vi "添加设备.vi"(7 "模式":enum16{"新建设备", "编辑设备"}(ring), 8 "错误输出":errorcluster, 11 "探头属性 i":T1) -> (0 "error out":errorcluster, 1 "附加信息":string, 2 "输出有效？":bool=TRUE, 3 "探头属性 o":T1)   [LabVIEW 2017]
doc: "修改信息时 : 输入完整信息 ,\n新建时 : 输入空常量 ."
uses:
  <vilib>/Utility/miscctls.llb/LVSelectionTypeDef.ctl
  df94b285-9738-4c66-b3c8-f98dc0b9297b.vi
  c5779a91-24a2-4c03-8a90-ef35a31279a1.vi
panel:
  out "改串口地址?":bool
  out "前缀":enum16{"Net", "Serial"}(ring)
  out "专用标志-首次 '端口值改变' 事件":bool=TRUE
  in  "设置系数":bool
  in  "类型":enum16{"网络探头", "串口探头"}(ring)
  in  "超时":i32
  out "已保存的探头号":u16[](array[numeric])
  in  "标题":string
  out "提示语 2":string
  in  "探头备注":string
  out "提示语":string
  in  "探头名称":string caption="探头名称 *"
  in  "取消":bool
  in  "确定":bool
  in  "地址":string caption="探头 *"
  in  "端口":u16 caption="探头号 *" min=1 max=255
  out "有效名称？":bool
  out "有效地址？":bool
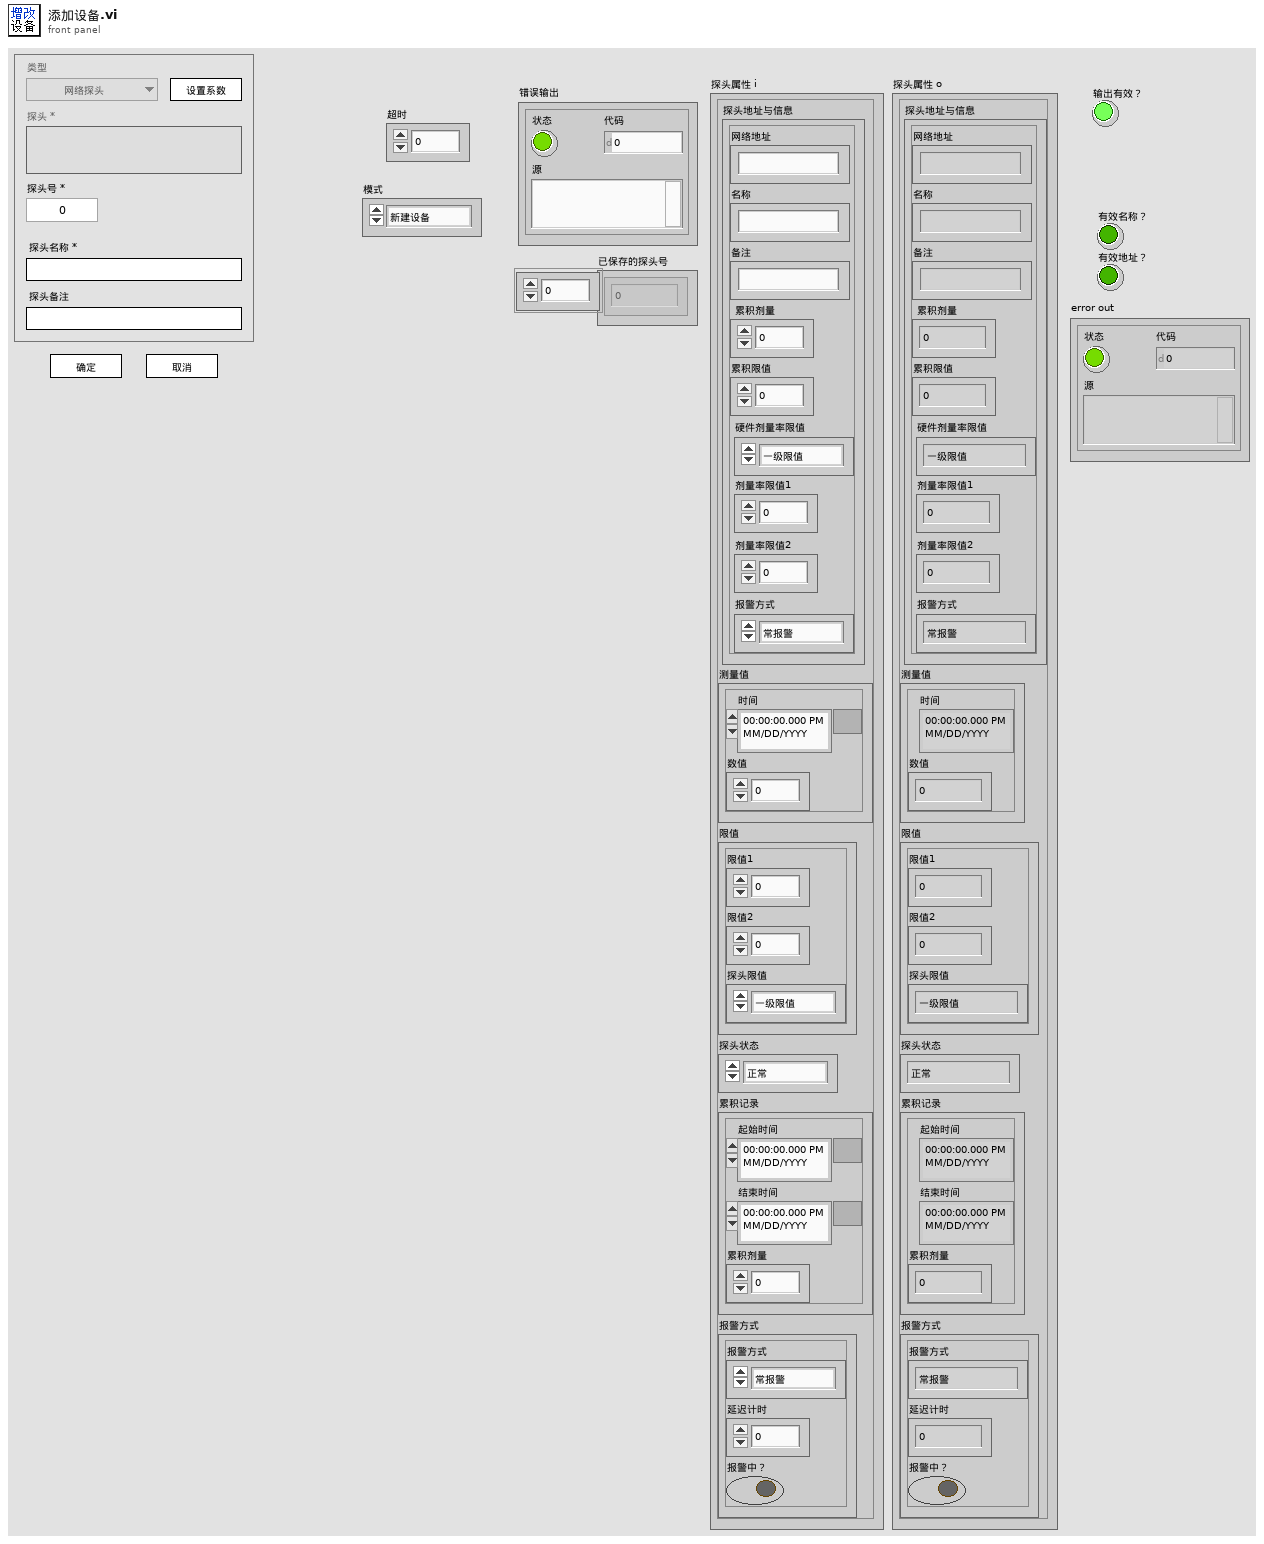
[diagram p1: front panel]
types:
  T1 = typedef "探头属性.ctl" = cluster{"探头地址与信息":T2, "测量值":T5, "限值":T6, "探头状态":T7, "累积记录":T8, "报警方式":T9}
  T2 = typedef "探测器信息.ctl" = cluster{"网络地址":string, "名称":string, "备注":string, "累积剂量":dbl, "累积限值":dbl, "硬件剂量率限值":T3, "剂量率限值1":dbl, "剂量率限值2":dbl, "报警方式":T4}
  T3 = typedef "探头剂量率限值选择.ctl" = enum16{"一级限值", "二级限值"}
  T4 = typedef "报警方式选择.ctl" = enum16{"常报警", "自动静音", "手动静音"}
  T5 = typedef "测量值.ctl" = cluster{"时间":timestamp, "数值":dbl}
  T6 = typedef "剂量率限值.ctl" = cluster{"限值1":dbl, "限值2":dbl, "探头限值":T3}
  T7 = typedef "探头状态.ctl" = enum16{"正常", "离线", "禁用", "一级报警", "二级报警", "累积报警"}
  T8 = typedef "单条累积记录.ctl" = cluster{"起始时间":timestamp, "结束时间":timestamp, "累积剂量":dbl}
  T9 = typedef "报警方式.ctl" = cluster{"报警方式":T4, "延迟计时":u16, "报警中？":bool}
  T10 = enum32{"Invalid", "Standard", "Closed", "Hidden", "Minimized", "Maximized"}
  T11 = typedef "DB动作与数据.ctl" = cluster{"动作类型":T12, "输入数据":variant}
  T12 = typedef "DB动作类型.ctl" = enum16{"DB-文件初始化+连接", "DB-断开连接", "DB-结构初始化", "DB-加载设备", "DB-检查连接状态", "设备-登记新设备+数据表", "设备-删除设备", "设备-修改网址", "设备-修改名称+转移数据", "设备-修改备注", "设备-修改限值", "设备-累积校准", "设备-重排", "数据-获取全部", "数据-删除数据", "数据-写改累积记录+改累积剂量", "读变量-全部设备"}
  T13 = typedef "串口配置.ctl" = cluster{"COM口":refnum<visa-resource-name>, "波特率":enum16{"9600", "19200"}, "探头地址(U8)":u8}
  T14 = typedef "探头系数.ctl" = cluster{"N1":u16, "N2":u16}
  T15 = typedef "串口模块输入.ctl" = cluster{"串口动作类型":T16, "串口配置":T13, "数据输入":variant}
  T16 = typedef "串口动作类型.ctl" = enum16{"读测量值", "设置报警值", "设置地址", "设置系数", "广播修改波特率", "关闭串口"}
  T17 = enum8{"Enabled", "Disabled", "Disabled and Grayed Out"}
  T18 = typedef "LVSelectionTypeDef.ctl" = cluster{"Selection Start":u32, "Selection End":u32}
  T19 = typedef "簇-输入.ctl" = cluster{"配置文件动作":T20, "数据输入":variant}
  T20 = typedef "枚举-配置文件动作.ctl" = enum16{"初始化加载配置", "读取配置", "写入-屏幕键盘", "写入-静音延迟", "写入-主要探头类型", "写入-串口配置", "写入-累积定时", "写入-导出定时", "保存配置到文件"}
  T21 = typedef "簇-配置文件内容.ctl" = cluster{"调试模式？":bool, "屏幕键盘？":bool, "软件版本":string, "静音延迟 s":u16, "主要探头类型":T22, "串口配置":cluster{"COM口":refnum<visa-resource-name>, "波特率":enum16{"9600", "19200"}, "读写超时ms":i16, "丢包判定次数":i16}, "定时配置-累积分段":T23, "定时配置-自动导出":cluster{"定时配置-自动导出":T23, "分别导出?":bool}}
  T22 = typedef "枚举-主要探头类型.ctl" = enum16{"网络探头", "串口探头"}
  T23 = typedef "簇-定时配置.ctl" = cluster{"定时模式":enum16{"绝对时间", "相对时间"}, "单位":enum16{"年", "月", "日", "时", "分"}, "间隔":u8, "目标时刻":timestamp}
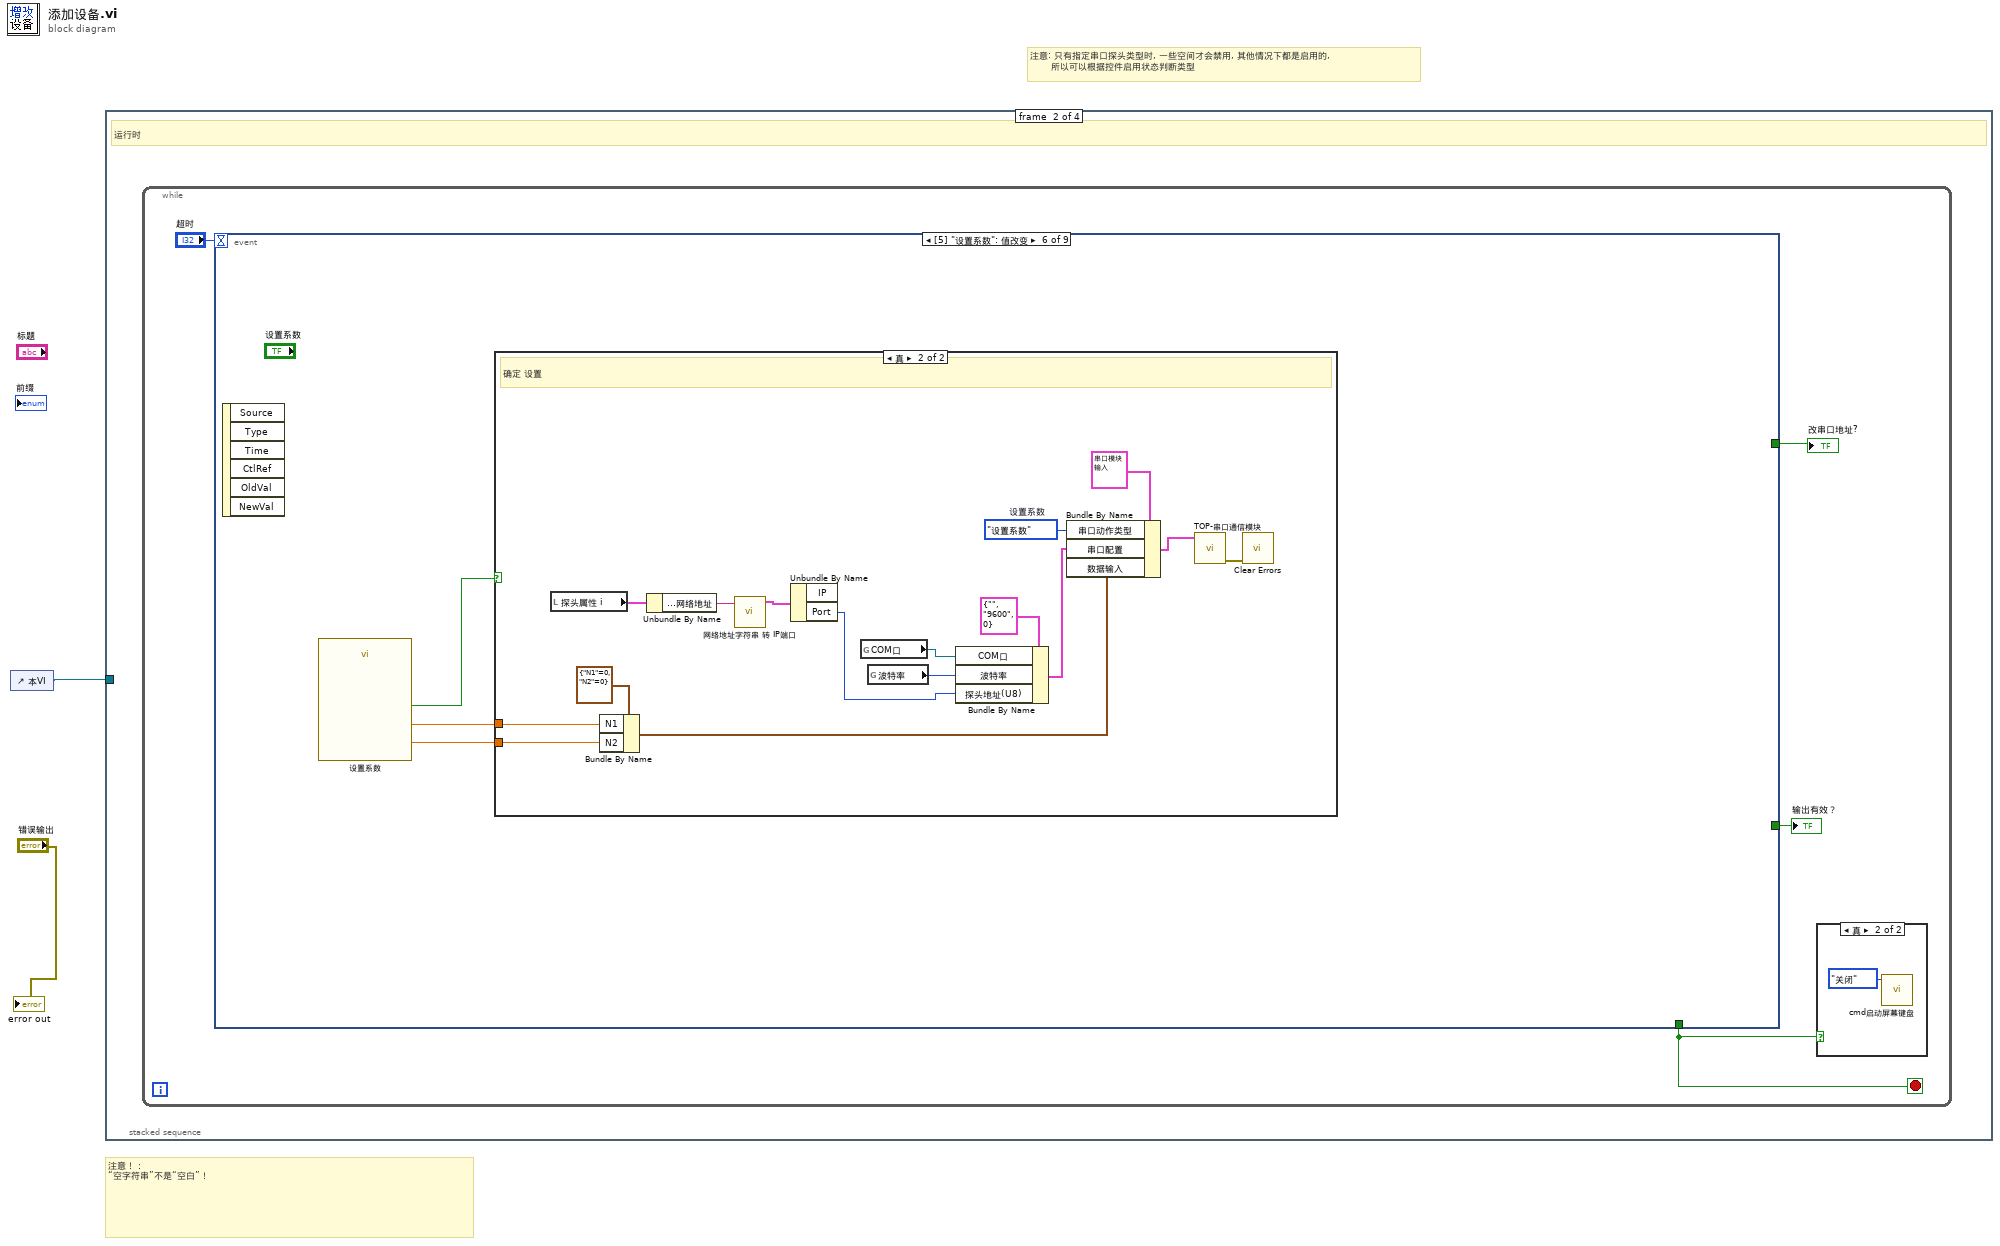
[diagram p0: block diagram]
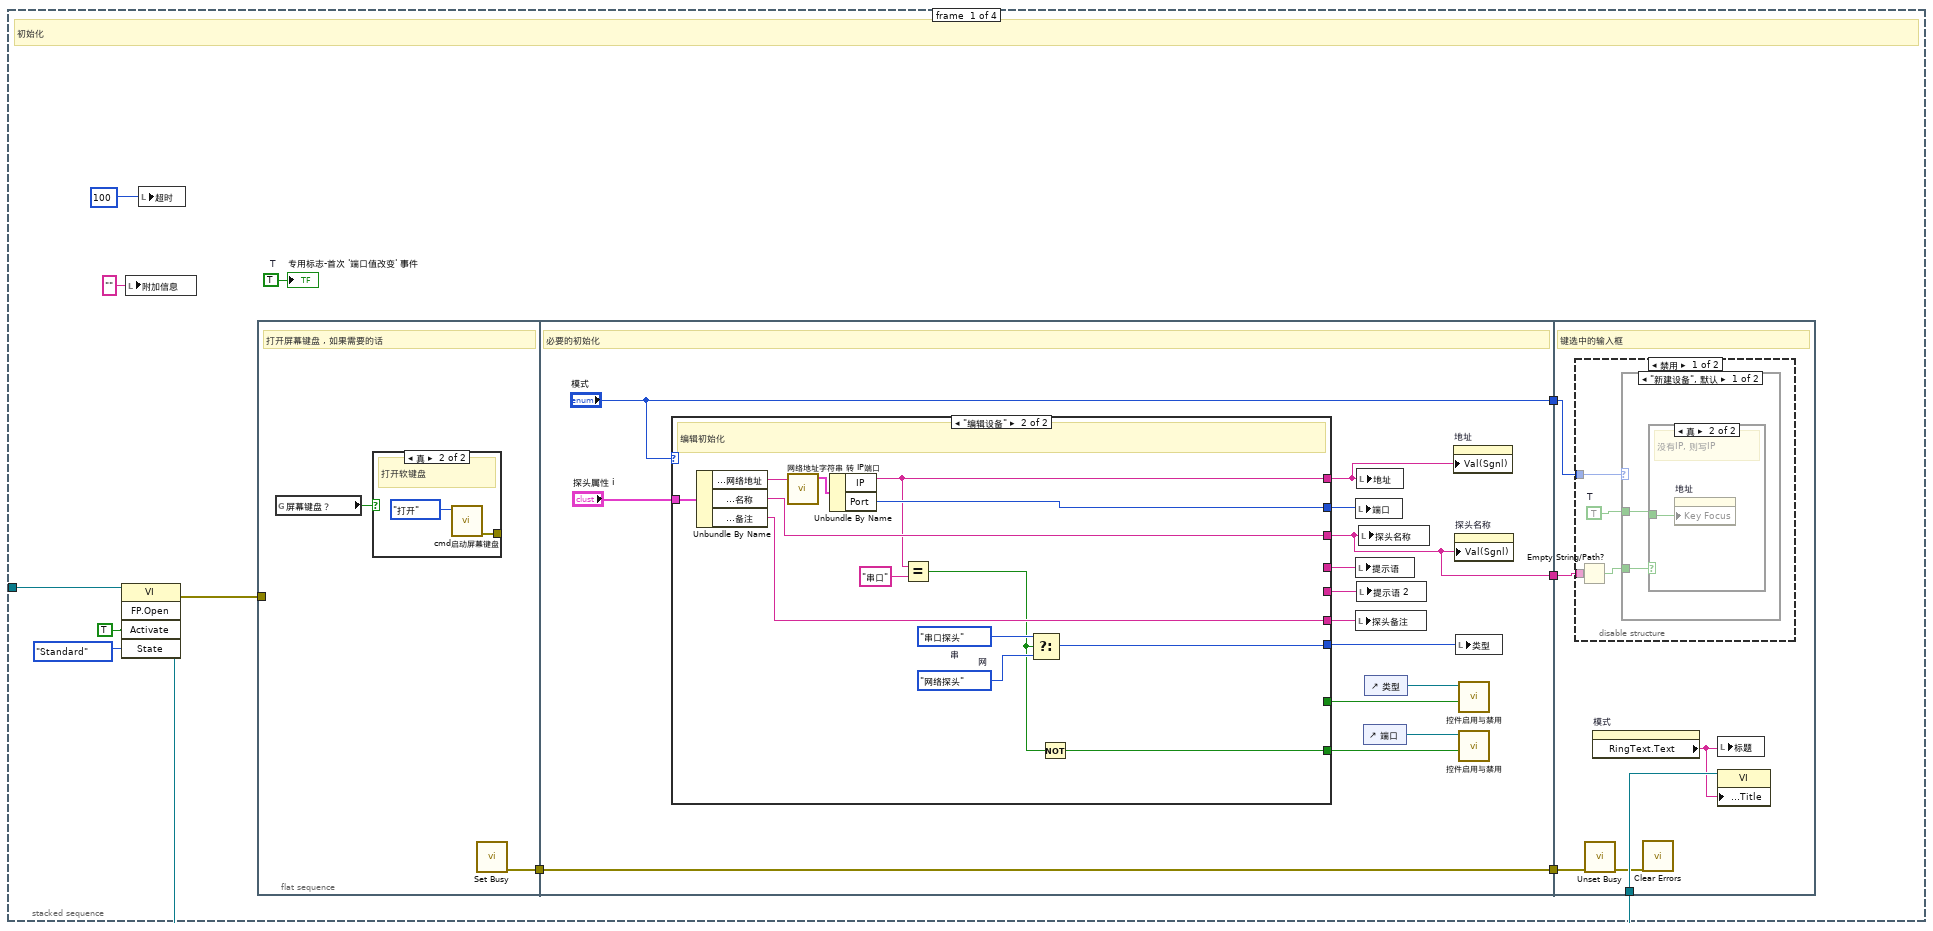
[diagram p2: hidden frame]
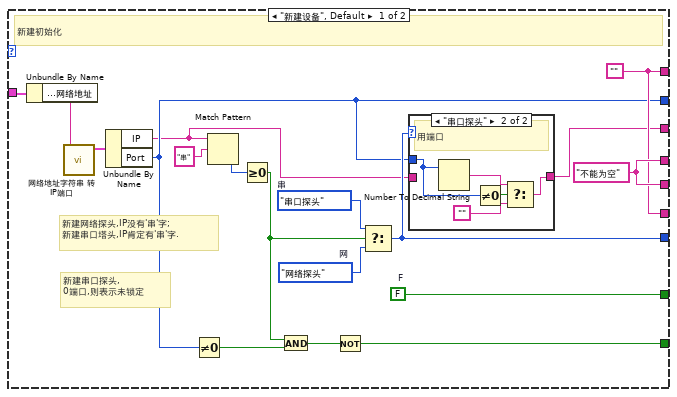
[diagram p4: hidden frame]
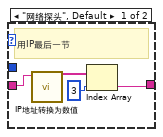
[diagram p5: hidden frame]
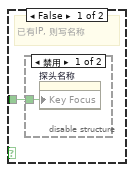
[diagram p6: hidden frame]
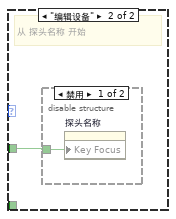
[diagram p8: hidden frame]
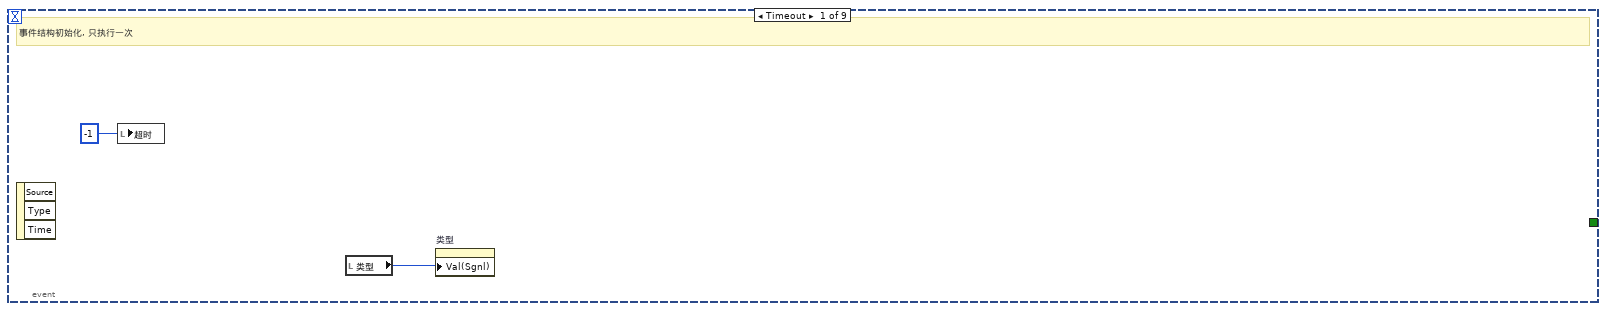
[diagram p12: hidden frame]
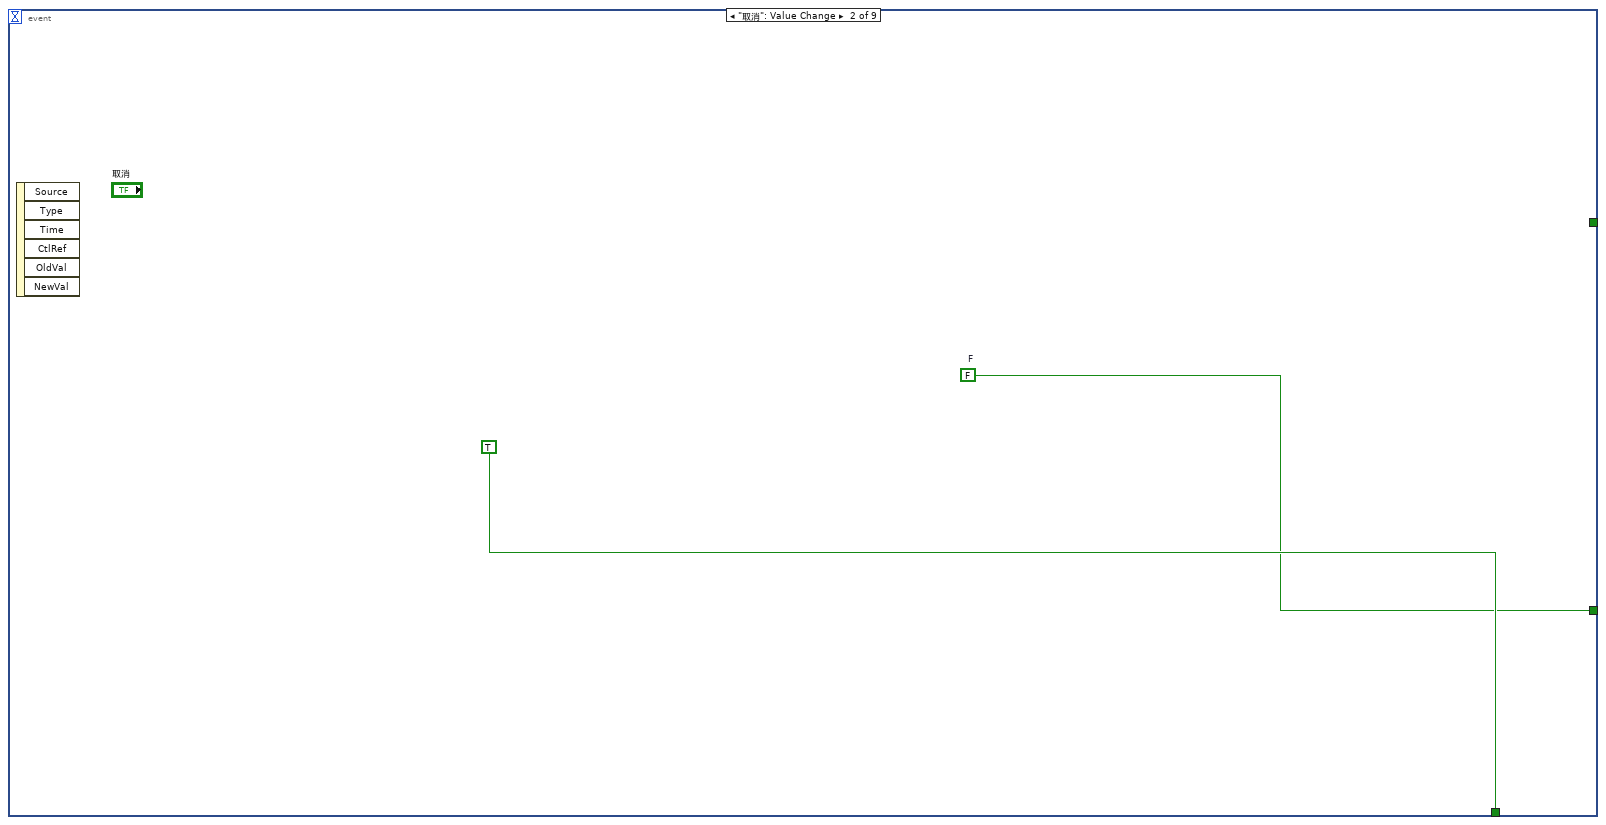
[diagram p13: hidden frame]
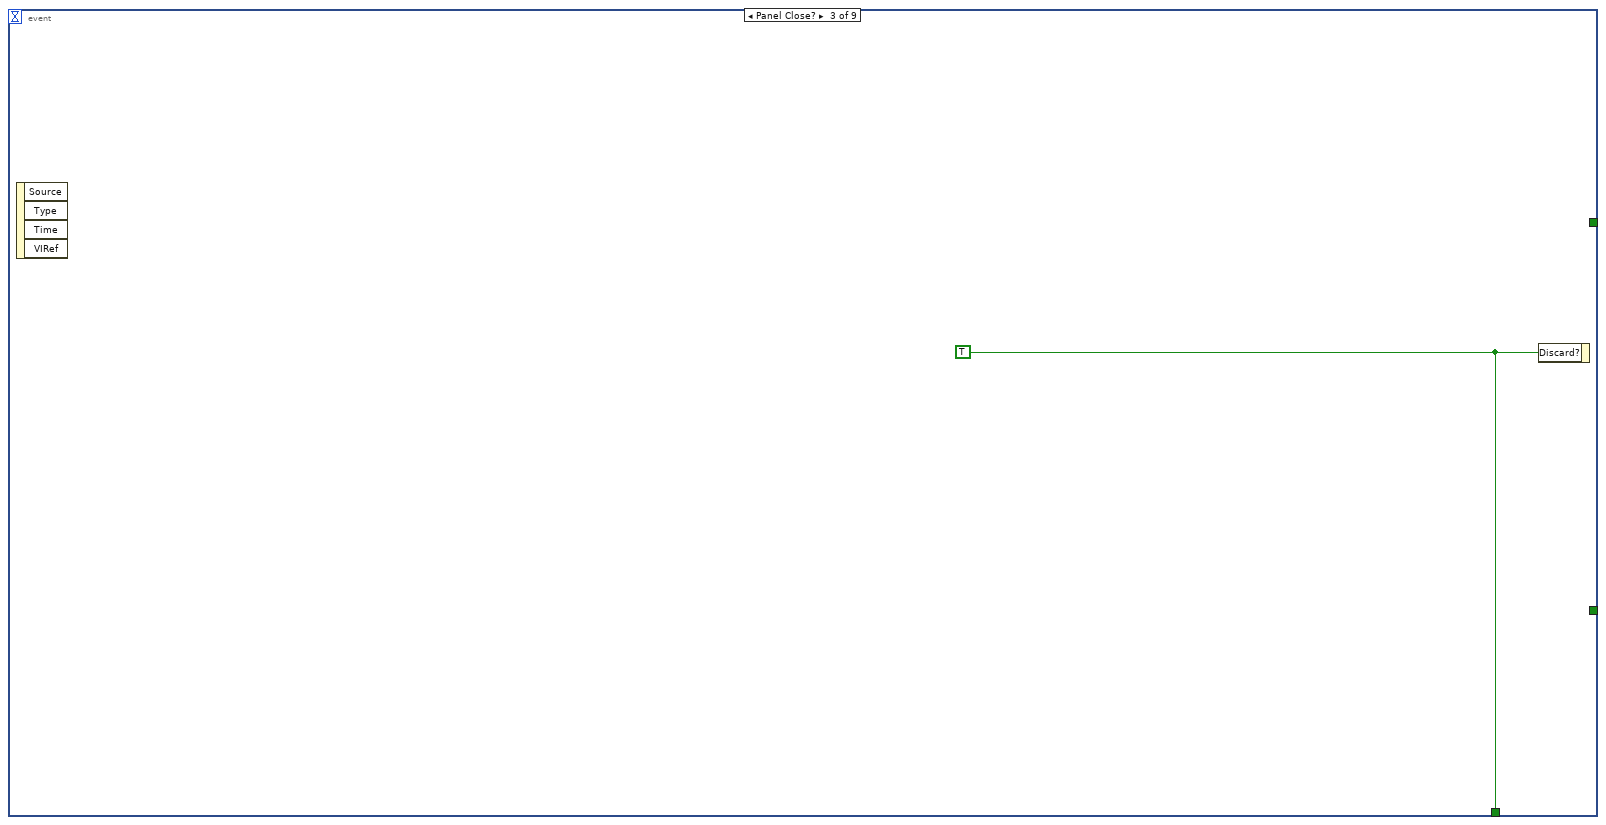
[diagram p14: hidden frame]
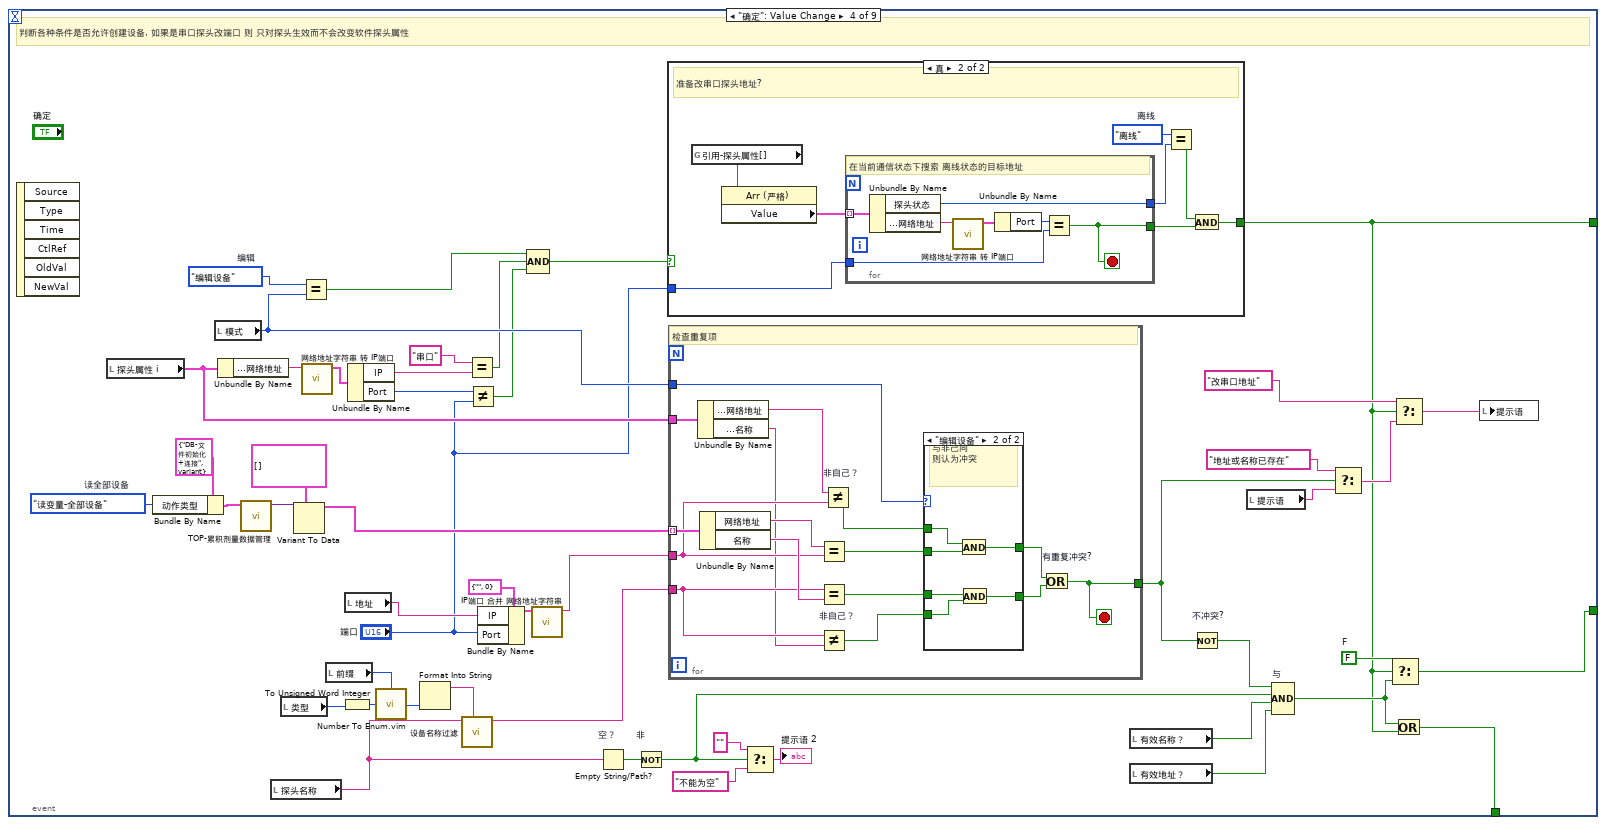
[diagram p15: hidden frame]
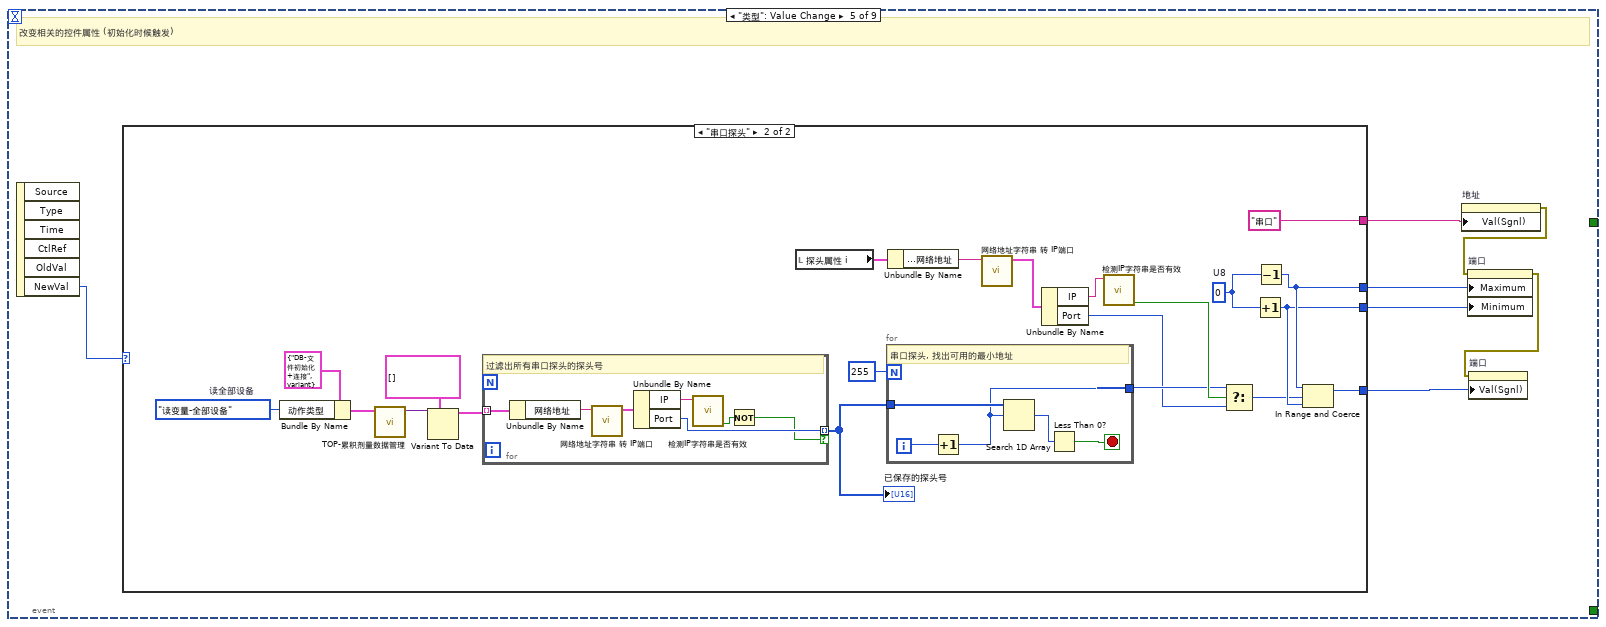
[diagram p18: hidden frame]
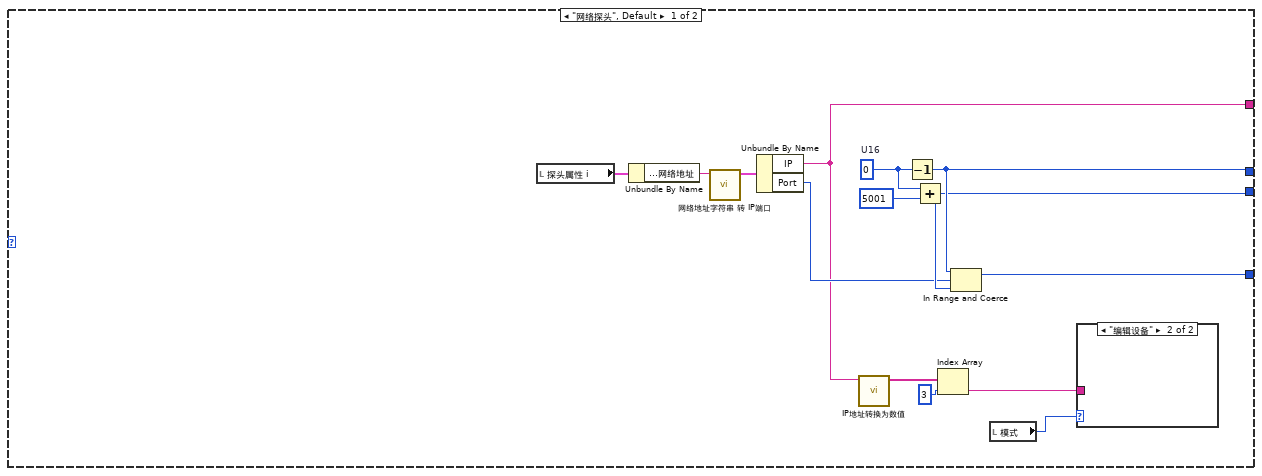
[diagram p19: hidden frame]
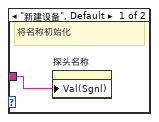
[diagram p20: hidden frame]
diagram:
  # "注意: 只有指定串口探头类型时, 一些空间才会禁用, 其他情况下都是启用的,\n       所以可以根据控件启用状态判断类型"
  # "注意！：\n“空字符串”不是“空白”！"
  n1 = control-ref of="本VI"() -> (w2:refnum<vi>)
  n2 = stacked-sequence {
    tunnel: w2 -> [w12 _ _ w415]
    frame #0 {
      w6 = TRUE  # T
      # "初始化"
      n3 = invoke class="VI" method="FP.Open"(reference=w12, "Activate"=TRUE ("激活？"), "State"=T10."Standard" ("状态")) -> (reference out=w9:refnum<vi>, error out=w10:errorcluster)  [unwired: 2 in, 3 out]
      n4 = local write "附加信息"("" ("附加信息")) -> ()
      n5 = local write "超时"(100 ("超时")) -> ()
      n6 = flat-sequence {
        tunnel: w10 -> [_]
        tunnel: [w15] -> w3
        tunnel: ["模式"] -> w11
        tunnel: [w20] -> w7
        tunnel: [w19] -> w4
        tunnel: w3 -> [w19]
        tunnel: w11 -> [w78]
        tunnel: w9 -> [w77]
        tunnel: w7 -> [w75]
        tunnel: w4 -> [w74]
        frame #0 {
          # "打开屏幕键盘 , 如果需要的话"
          n7 = global read "全局变量-35点监测.vi" "屏幕键盘？"() -> (w16:bool)
          n8 = case shown="真" w16 {
            tunnel: [_ w17] -> _
            frame False {
            }
            frame True {
              # "打开软键盘"
              n9 = call "cmd启动屏幕键盘.vi"("软键盘开关"=enum16{"关闭", "打开"}."打开") -> ("error out"=w17:errorcluster)  [unwired: 9 in, 1 out]
            }
          }
          n10 = call <vilib>:"Set Busy.vi"() -> ("error out"=w15:errorcluster)  [unwired: 10 in, 1 out]
        }
        frame #1 {
          # "必要的初始化"
          n11 = case shown="\"编辑设备\"" "模式" {
            tunnel: [w49 w66] -> w28
            tunnel: [w35 w69] -> w32
            tunnel: [w50 _] -> w31
            tunnel: [w50 _] -> w30
            tunnel: [w34 w68] -> w20
            tunnel: "探头属性 i" -> [w48 w72]
            tunnel: [w49 w67] -> w27
            tunnel: [w40 _] -> w23
            tunnel: [w41 w60] -> w22
            tunnel: [w36 w62] -> w21
            frame "新建设备", Default {
              w40 = FALSE  # F
              w42 = enum16{"网络探头", "串口探头"}."网络探头"  # 网
              w43 = enum16{"网络探头", "串口探头"}."串口探头"  # 串
              w50 = "不能为空" ("探头名称")
              w49 = ""
              # "新建串口探头, \n0端口,则表示未锁定"
              # "新建网络探头,IP没有'串'字;\n新建串口塔头,IP肯定有'串'字."
              # "新建初始化"
              n12 = Unbundle By Name(w48) -> ("探头地址与信息.网络地址"=w46:string)
              n13 = call "网络地址字符串 转 IP端口.vi"("IP端口字符串"=w46) -> ("IP端口"=w47:cluster{"IP":string, "Port":u16})  [unwired: 10 in]
              n14 = Unbundle By Name(w47) -> ("IP"=w33:string, "Port"=w35:u16)
              n15 = Not Equal To 0?(x=w35) -> (x != 0?=w45:bool)
              n16 = Match Pattern(string=w33, regular expression="串" ("正则表达式")) -> (offset past match=w38:i32)  [unwired: 1 in, 3 out]
              n17 = Greater Or Equal To 0?(x=w38) -> (x >= 0?=w37:bool)
              n18 = And(x=w37, y=w45) -> (x .and. y?=w44:bool)
              n19 = Not(x=w44) -> (.not. x?=w41:bool)
              n20 = Select(t=w43, s=w37, f=w42) -> (s? t:f=w36:enum16{"网络探头", "串口探头"})
              n21 = case shown="\"串口探头\"" w36 {
                tunnel: w35 -> [_ w59]
                tunnel: [w51 w55] -> w34
                tunnel: w33 -> [w54 _]
                frame "网络探头", Default {
                  # "用IP最后一节"
                  n22 = call "IP地址转换为数值.vi"("IP地址"=w54) -> ("字符串数组"=w53:string[])  [unwired: 8 in, 2 out]
                  n23 = Index Array(array=w53, index=3 ("索引")) -> (element=w51:string)
                }
                frame "串口探头" {
                  # "用端口"
                  n24 = Number To Decimal String(number=w59) -> (decimal integer string=w56:string)  [unwired: 1 in]
                  n25 = Not Equal To 0?(x=w59) -> (x != 0?=w58:bool)
                  n26 = Select(t=w56, s=w58, f="") -> (s? t:f=w55:string)
                }
              }
            }
            frame "编辑设备" {
              w64 = enum16{"网络探头", "串口探头"}."串口探头"  # 串
              w63 = enum16{"网络探头", "串口探头"}."网络探头"  # 网
              # "编辑初始化"
              n27 = Unbundle By Name(w72) -> ("探头地址与信息.网络地址"=w71:string, "探头地址与信息.名称"=w68:string, "探头地址与信息.备注"=w67:string)
              n28 = call "网络地址字符串 转 IP端口.vi"("IP端口字符串"=w71) -> ("IP端口"=w70:cluster{"IP":string, "Port":u16})  [unwired: 10 in]
              n29 = Unbundle By Name(w70) -> ("IP"=w66:string, "Port"=w69:u16)
              n30 = Equal?(x=w66, y="串口") -> (x = y?=w61:bool)
              n31 = Select(t=w64, s=w61, f=w63) -> (s? t:f=w62:enum16{"网络探头", "串口探头"})
              n32 = Not(x=w61) -> (.not. x?=w60:bool)
            }
          }
          n33 = local write "端口"(w32) -> ()
          n34 = local write "提示语"(w31) -> ()
          n35 = local write "探头备注"(w27) -> ()
          n36 = local write "地址"(w28) -> ()
          n37 = local write "提示语 2"(w30) -> ()
          n38 = local write "探头名称"(w20) -> ()
          n39 = control-ref of="端口"() -> (w25:refnum<vi>)
          n40 = control-ref of="类型"() -> (w24:refnum<vi>)
          n41 = property on="地址" class="Str"("Val(Sgnl)"=w28) -> ()  [unwired: 2 in, 2 out]
          n42 = property on="探头名称" class="Str"("Val(Sgnl)"=w20) -> ()  [unwired: 2 in, 2 out]
          n43 = local write "类型"(w21) -> ()
          n44 = call "控件启用与禁用.vi"("启用？"=w23, "控件引用"=w24) -> ()  [unwired: 9 in, 1 out]
          n45 = call "控件启用与禁用.vi"("启用？"=w22, "控件引用"=w25) -> ()  [unwired: 9 in, 1 out]
        }
        frame #2 {
          # "键选中的输入框"
          n46 = disable-structure shown="禁用" {
            disable-tunnel: w78 -> [w82 _]
            disable-tunnel: w75 -> [w80 _]
            frame Disabled {
              w81 = TRUE  # T
              n47 = Empty String/Path?(string/path=w80) -> (empty?=w79:bool)
              n48 = case shown="\"新建设备\", 默认" w82 {
                tunnel: w81 -> [w84 w88]
                tunnel: w79 -> [w83 _]
                frame "新建设备", Default {
                  n49 = case shown="真" w83 {
                    tunnel: w84 -> [w85 w87]
                    frame False {
                      # "已有IP, 则写名称"
                      n50 = disable-structure shown="禁用" {
                        disable-tunnel: w85 -> [w86 _]
                        frame Disabled {
                          n51 = property on="探头名称" class="Str"("Key Focus"=w86) -> ()  [unwired: 2 in, 2 out]
                        }
                        frame Enabled {
                        }
                      }
                    }
                    frame True {
                      # "没有IP, 则写IP"
                      n52 = property on="地址" class="Str"("Key Focus"=w87) -> ()  [unwired: 2 in, 2 out]
                    }
                  }
                }
                frame "编辑设备" {
                  # "从 探头名称 开始"
                  n53 = disable-structure shown="禁用" {
                    disable-tunnel: w88 -> [w89 _]
                    frame Disabled {
                      n54 = property on="探头名称" class="Str"("Key Focus"=w89) -> ()  [unwired: 2 in, 2 out]
                    }
                    frame Enabled {
                    }
                  }
                }
              }
            }
            frame Enabled {
            }
          }
          n55 = call <vilib>:"Unset Busy.vi"("error in (no error)"=w74) -> ("error out"=w73:errorcluster)  [unwired: 10 in]
          n56 = property on="模式" class="枚举 (严格)"() -> ("RingText.Text"=w76:string)  [unwired: 2 in, 2 out]
          n57 = call <vilib>:"Clear Errors.vi"("error in (no error)"=w73) -> ()  [unwired: 5 in, 2 out]
          n58 = local write "标题"(w76) -> ()
          n59 = property class="VI"(reference=w77, "Front Panel.Title"=w76) -> ()  [unwired: 1 in, 2 out]
        }
      }
      "专用标志-首次 '端口值改变' 事件" <- w6
    }
    frame #1 {
      # "运行时"
      n60 = while {
        stop <- w92 stop-if-true
        n61 = event shown="[5] \"设置系数\": 值改变" {
          selector: _ -> [_ _ _ _ _ _ _ _ _]
          dyn-events: _ -> [_ _ _ _ _ _ _ _ _]
          timeout: "超时" -> [_ _ _ _ _ _ _ _ _]
          tunnel: [_ TRUE ("放弃？") w99 w101 _ _ _ _ _] -> w92
          tunnel: [_ w97 _ w102 _ _ _ _ _] -> w93
          tunnel: [_ _ _ w100 _ _ _ _ _] -> w90
          event Timeout {
            # "事件结构初始化, 只执行一次"
            n62 = event-data() -> ()  [unwired: 1 in, 3 out]
            n63 = local write "超时"(-1 ("超时")) -> ()
            n64 = local read "类型"() -> (w95:enum16{"网络探头", "串口探头"})
            n65 = property on="类型" class="Enum (严格)"("Val(Sgnl)"=w95) -> ()  [unwired: 2 in, 2 out]
          }
          event "取消": Value Change {
            w97 = FALSE  # F
            n66 = event-data() -> ()  [unwired: 1 in, 6 out]
          }
          event Panel Close? {
            w99 = TRUE ("放弃？")
            n67 = event-data() -> ()  [unwired: 1 in, 4 out]
            n68 = event-data("Discard?"=w99) -> ()  [unwired: 1 in, 1 out]
          }
          event "确定": Value Change {
            w104 = FALSE  # F
            w121 = enum16{"新建设备", "编辑设备"}."编辑设备"  # 编辑
            w132 = DB动作类型."读变量-全部设备"  # 读全部设备
            # "判断各种条件是否允许创建设备, 如果是串口探头改端口 则 只对探头生效而不会改变软件探头属性"
            n69 = event-data() -> ()  [unwired: 1 in, 6 out]
            n70 = local read "探头属性 i"() -> (w118:T1)
            n71 = Bundle By Name(cluster=T11 {"动作类型"=enum."DB-文件初始化+连接", "输入数据"=variant} ("DB动作集"), "动作类型"=w132) -> (w131:T11)
            n72 = local read "模式"() -> (w122:enum16{"新建设备", "编辑设备"})
            n73 = Unbundle By Name(w118) -> ("探头地址与信息.网络地址"=w117:string)
            n74 = call "TOP-累积剂量数据管理.vi"("DB动作集"=w131) -> ("输出数据"=w130:variant)  [unwired: 9 in, 1 out]
            n75 = local read "探头名称"() -> (w124:string)
            n76 = local read "类型"() -> (w120:enum16{"网络探头", "串口探头"})
            n77 = Variant To Data(type=T2[] [] ("探测器清单"), Variant=w130) -> (data=w110:T2[])  [unwired: 1 in, 1 out]
            n78 = Equal?(x=w121, y=w122) -> (x = y?=w113:bool)
            n79 = call "网络地址字符串 转 IP端口.vi"("IP端口字符串"=w117) -> ("IP端口"=w119:cluster{"IP":string, "Port":u16})  [unwired: 10 in]
            n80 = local read "前缀"() -> (w125:enum16{"Net", "Serial"})
            n81 = To Unsigned Word Integer(number=w120) -> (unsigned 16bit integer=w126:u16)
            n82 = local read "地址"() -> (w145:string)
            n83 = Unbundle By Name(w119) -> ("IP"=w116:string, "Port"=w114:u16)
            n84 = call "Number To Enum.vim"("number"=w126, "enum type"=w125) -> ("number as enum"=w127:enum16{"Net", "Serial"})
            n85 = Format Into String(w127) -> (resulting string=w128:string)  [unwired: 3 in, 1 out]
            n86 = call "设备名称过滤.vi"("前缀"=w128, "字符串 i"=w124) -> ("字符串 o"=w123:string)  [unwired: 9 in]
            n87 = Equal?(x="串口", y=w116) -> (x = y?=w112:bool)
            n88 = Not Equal?(x=w114, y="端口") -> (x != y?=w111:bool)
            n89 = Bundle By Name(cluster=cluster{"IP":string, "Port":u16} {"IP"="", "Port"=0} ("IP端口"), "IP"=w145, "Port"="端口") -> (w146:cluster{"IP":string, "Port":u16})
            n90 = Compound Arithmetic op=AND ("复合运算")(w113, w112, w111) -> (w109:bool)
            n91 = call "IP端口 合并 网络地址字符串.vi"("IP端口"=w146) -> ("IP端口字符串"=w144:string)  [unwired: 10 in]
            n92 = Empty String/Path? "空？"(string/path=w124) -> (empty?=w148:bool)
            n93 = Not "非"(x=w148) -> (.not. x?=w136:bool)
            n94 = case shown="真" w109 {
              tunnel: "端口" -> [_ w154]
              tunnel: [_ w150] -> w100
              frame False {
              }
              frame True {
                w151 = 探头状态."离线"  # 离线
                # "准备改串口探头地址?"
                n95 = global read "全局变量-35点监测.vi" "引用-探头属性[]"() -> (w156:refnum<vi>)
                n96 = property class="Arr (严格)"(reference=w156) -> ("Value"=w155:T1[])  [unwired: 1 in, 2 out]
                n97 = for {
                  tunnel: w155 -> [w161] mode=indexing
                  tunnel: [w159] -> w153
                  tunnel: w154 -> [w158]
                  tunnel: [w157] -> w152
                  stop <- w159 stop-if-true
                  # "在当前通信状态下搜索 离线状态的目标地址"
                  n98 = Unbundle By Name(w161) -> ("探头状态"=w157:T7, "探头地址与信息.网络地址"=w162:string)
                  n99 = call "网络地址字符串 转 IP端口.vi"("IP端口字符串"=w162) -> ("IP端口"=w163:cluster{"IP":string, "Port":u16})  [unwired: 10 in]
                  n100 = Unbundle By Name(w163) -> ("Port"=w160:u16)
                  n101 = Equal?(x=w160, y=w158) -> (x = y?=w159:bool)
                }
                n102 = Equal?(x=w151, y=w152) -> (x = y?=w149:bool)
                n103 = And(x=w149, y=w153) -> (x .and. y?=w150:bool)
              }
            }
            n104 = for {
              tunnel: w110 -> [w179] mode=indexing
              tunnel: w144 -> [w170]
              tunnel: w123 -> [w168]
              tunnel: [w174] -> w138
              tunnel: w118 -> [w173]
              tunnel: w122 -> [w164]
              stop <- w174 stop-if-true
              # "检查重复项"
              n105 = Unbundle By Name(w173) -> ("探头地址与信息.网络地址"=w169:string, "探头地址与信息.名称"=w167:string)
              n106 = Unbundle By Name(w179) -> ("网络地址"=w178:string, "名称"=w177:string)
              n107 = Equal?(x=w178, y=w170) -> (x = y?=w176:bool)
              n108 = Equal?(x=w168, y=w177) -> (x = y?=w175:bool)
              n109 = Not Equal? "非自己？"(x=w168, y=w167) -> (x != y?=w165:bool)
              n110 = Not Equal? "非自己？"(x=w169, y=w170) -> (x != y?=w166:bool)
              n111 = case shown="\"编辑设备\"" w164 {
                tunnel: w176 -> [w181 w187]
                tunnel: w175 -> [w180 w186]
                tunnel: [w181 w185] -> w172
                tunnel: [w180 w184] -> w171
                tunnel: w166 -> [_ w183]
                tunnel: w165 -> [_ w182]
                frame "新建设备", Default {
                  # "有相同\n则认为冲突"
                }
                frame "编辑设备" {
                  # "与非己同\n则认为冲突"
                  n112 = And(x=w183, y=w187) -> (x .and. y?=w185:bool)
                  n113 = And(x=w186, y=w182) -> (x .and. y?=w184:bool)
                }
              }
              n114 = Or "有重复冲突?"(x=w172, y=w171) -> (x .or. y?=w174:bool)
            }
            n115 = Select(t="", s=w136, f="不能为空") -> (s? t:f=→"提示语 2":string)
            n116 = local read "有效名称？"() -> (w135:bool)
            n117 = local read "有效地址？"() -> (w134:bool)
            n118 = Not "不冲突?"(x=w138) -> (.not. x?=w137:bool)
            n119 = local read "提示语"() -> (w140:string)
            n120 = Compound Arithmetic op=AND "与"(w137, w136, w135, w134) -> (w103:bool)
            n121 = Select(t="地址或名称已存在", s=w138, f=w140) -> (s? t:f=w106:string)
            n122 = Select(t=w104, s=w100, f=w103) -> (s? t:f=w102:bool)
            n123 = Select(t="改串口地址", s=w100, f=w106) -> (s? t:f=w105:string)
            n124 = Or(x=w103, y=w100) -> (x .or. y?=w101:bool)
            n125 = local write "提示语"(w105) -> ()
          }
          event "类型": Value Change {
            # "改变相关的控件属性 (初始化时候触发)"
            n126 = event-data() -> ("NewVal"=w194:enum16{"网络探头", "串口探头"})  [unwired: 1 in, 5 out]
            n127 = case shown="\"串口探头\"" w194 {
              tunnel: [w198 "串口"] -> w193
              tunnel: [w200 w210] -> w192
              tunnel: [w203 w213] -> w190
              tunnel: [w202 w212] -> w189
              frame "网络探头", Default {
                w204 = u16 0  # U16
                n128 = local read "探头属性 i"() -> (w208:T1)
                n129 = Unbundle By Name(w208) -> ("探头地址与信息.网络地址"=w206:string)
                n130 = call "网络地址字符串 转 IP端口.vi"("IP端口字符串"=w206) -> ("IP端口"=w207:cluster{"IP":string, "Port":u16})  [unwired: 10 in]
                n131 = Unbundle By Name(w207) -> ("IP"=w198:string, "Port"=w201:u16)
                n132 = call "IP地址转换为数值.vi"("IP地址"=w198) -> ("字符串数组"=w197:string[])  [unwired: 8 in, 2 out]
                n133 = Decrement(x=w204) -> (x-1=w203:u16)
                n134 = Add(x=w204, y=u16 5001 ("x")) -> (x+y=w202:u16)
                n135 = Index Array(array=w197, index=3 ("索引")) -> (element=w195:string)
                n136 = In Range and Coerce(upper limit=w203, x=w201, lower limit=w202) -> (coerced(x)=w200:u16)  [unwired: 1 out]
                n137 = local read "模式"() -> (w196:enum16{"新建设备", "编辑设备"})
                n138 = case shown="\"编辑设备\"" w196 {
                  tunnel: w195 -> [w209 _]
                  frame "新建设备", Default {
                    # "将名称初始化"
                    n139 = property on="探头名称" class="Str"("Val(Sgnl)"=w209) -> ()  [unwired: 2 in, 2 out]
                  }
                  frame "编辑设备" {
                  }
                }
              }
              frame "串口探头" {
                w214 = u8 0  # U8
                w225 = DB动作类型."读变量-全部设备"  # 读全部设备
                n140 = Bundle By Name(cluster=T11 {"动作类型"=enum."DB-文件初始化+连接", "输入数据"=variant} ("DB动作集"), "动作类型"=w225) -> (w229:T11)
                n141 = call "TOP-累积剂量数据管理.vi"("DB动作集"=w229) -> ("输出数据"=w228:variant)  [unwired: 9 in, 1 out]
                n142 = Variant To Data(type=T2[] [] ("探测器清单"), Variant=w228) -> (data=w230:T2[])  [unwired: 1 in, 1 out]
                n143 = for {
                  tunnel: w230 -> [w242] mode=indexing
                  tunnel: [w238] -> w223 mode=indexing if=w236
                  # "过滤出所有串口探头的探头号"
                  n144 = Unbundle By Name(w242) -> ("网络地址"=w240:string)
                  n145 = call "网络地址字符串 转 IP端口.vi"("IP端口字符串"=w240) -> ("IP端口"=w241:cluster{"IP":string, "Port":u16})  [unwired: 10 in]
                  n146 = Unbundle By Name(w241) -> ("IP"=w239:string, "Port"=w238:u16)
                  n147 = call "检测IP字符串是否有效.vi"("IP地址"=w239) -> ("有效IP？"=w237:bool)  [unwired: 10 in]
                  n148 = Not(x=w237) -> (.not. x?=w236:bool)
                }
                "已保存的探头号" <- w223
                n149 = local read "探头属性 i"() -> (w221:T1)
                n150 = for {
                  N: 255 -> [_]
                  tunnel: w223 -> [w234]
                  tunnel: [w231] -> w216
                  i -> [w235]
                  stop <- w232 stop-if-true
                  # "串口探头, 找出可用的最小地址"
                  n151 = Increment(x=w235) -> (x+1=w231:i32)
                  n152 = Search 1D Array(1D array=w234, element=w231) -> (index of element=w233:i32)  [unwired: 1 in]
                  n153 = Less Than 0?(x=w233) -> (x < 0?=w232:bool)
                }
                n154 = Unbundle By Name(w221) -> ("探头地址与信息.网络地址"=w219:string)
                n155 = call "网络地址字符串 转 IP端口.vi"("IP端口字符串"=w219) -> ("IP端口"=w220:cluster{"IP":string, "Port":u16})  [unwired: 10 in]
                n156 = Unbundle By Name(w220) -> ("IP"=w218:string, "Port"=w215:u16)
                n157 = call "检测IP字符串是否有效.vi"("IP地址"=w218) -> ("有效IP？"=w217:bool)  [unwired: 10 in]
                n158 = Select(t=w216, s=w217, f=w215) -> (s? t:f=w211:i32)
                n159 = Increment(x=w214) -> (x+1=w212:u8)
                n160 = Decrement(x=w214) -> (x-1=w213:u8)
                n161 = In Range and Coerce(upper limit=w213, x=w211, lower limit=w212) -> (coerced(x)=w210:i32)  [unwired: 1 out]
              }
            }
            n162 = property on="地址" class="Str"("Val(Sgnl)"=w193) -> (error out=w188:errorcluster)  [unwired: 2 in, 1 out]
            n163 = property on="端口" class="DigNum (严格)"(error in=w188, "Maximum"=w190, "Minimum"=w189) -> (error out=w191:errorcluster)  [unwired: 1 in, 1 out]
            n164 = property on="端口" class="DigNum (严格)"(error in=w191, "Val(Sgnl)"=w192) -> ()  [unwired: 1 in, 2 out]
          }
          event "设置系数": Value Change {
            n165 = event-data() -> ()  [unwired: 1 in, 6 out]
            n166 = call "设置系数"() -> ("N2"=w244:dbl, "N1"=w245:dbl, "确定"=w243:bool)  [unwired: 16 in, 1 out]
            n167 = case shown="真" w243 {
              tunnel: w245 -> [_ w257]
              tunnel: w244 -> [_ w256]
              frame False {
                # "取消设置"
              }
              frame True {
                w259 = 串口动作类型."设置系数"  # 设置系数
                # "确定 设置"
                n168 = local read "探头属性 i"() -> (w253:T1)
                n169 = Bundle By Name(cluster=T14 {"N1"=0, "N2"=0}, "N1"=w257, "N2"=w256) -> (w247:T14)
                n170 = Unbundle By Name(w253) -> ("探头地址与信息.网络地址"=w255:string)
                n171 = call "网络地址字符串 转 IP端口.vi"("IP端口字符串"=w255) -> ("IP端口"=w254:cluster{"IP":string, "Port":u16})  [unwired: 10 in]
                n172 = Unbundle By Name(w254) -> ("Port"=w248:u16)  [unwired: 1 out]
                n173 = global read "全局变量-35点监测.vi" "COM口"() -> (w250:refnum<visa-resource-name>)
                n174 = global read "全局变量-35点监测.vi" "波特率"() -> (w249:enum16{"9600", "19200"})
                n175 = Bundle By Name(cluster=T13 {"COM口"="", "波特率"=enum."9600", "探头地址(U8)"=0} ("串口配置"), "COM口"=w250, "波特率"=w249, "探头地址(U8)"=w248) -> (w251:T13)
                n176 = Bundle By Name(cluster=T15 {"串口动作类型"=enum."读测量值", "串口配置"={"COM口"="", "波特率"=enum."9600", "探头地址(U8)"=0}, "数据输入"=variant} ("串口模块输入"), "串口动作类型"=w259, "串口配置"=w251, "数据输入"=w247) -> (w260:T15)
                n177 = call "TOP-串口通信模块.vi"("串口模块输入"=w260) -> ("error out"=w246:errorcluster)  [unwired: 9 in, 1 out]
                n178 = call <vilib>:"Clear Errors.vi"("error in (no error)"=w246) -> ()  [unwired: 5 in, 2 out]
              }
            }
          }
          event "地址": Value Change {
            # "实时检查地址格式，IP地址优先"
            n179 = event-data() -> ("NewVal"=w262:string)  [unwired: 1 in, 5 out]
            n180 = local read "类型"() -> (w265:enum16{"网络探头", "串口探头"})
            n181 = case shown="\"串口探头\"" w265 {
              tunnel: w262 -> [w280 _]
              tunnel: [w274 "串口探头"] -> w268
              tunnel: [w271 w283] -> w266
              tunnel: ["IP地址 *" ("标题.文本") "探头 *" ("标题.文本")] -> w264
              tunnel: [T17."Enabled" ("禁用") T17."Disabled and Grayed Out" ("禁用")] -> w263
              frame "网络探头", Default {
                # "地址判断"
                n182 = call <vilib>:"Trim Whitespace.vi"("string"=w280) -> ("trimmed string"=w273:string)  [unwired: 1 in]
                n183 = call "检测IP字符串是否有效.vi"("IP地址"=w273) -> ("有效IP？"=w279:bool)  [unwired: 10 in]
                n184 = call "字符串过滤-域名.vi"("字符串i"=w273) -> ("域名?"=w272:bool)  [unwired: 9 in, 1 out]
                n185 = Compound Arithmetic op=OR "或"(w272, w279) -> (w271:bool)
                n186 = Select(t="域名格式", s=w271, f="无效格式") -> (s? t:f=w275:string)
                n187 = Select(t="IP地址格式", s=w279, f=w275) -> (s? t:f=w274:string)
              }
              frame "串口探头" {
                w283 = TRUE  # T
                # "不需要判断"
              }
            }
            "提示语" <- w268
            "有效地址？" <- w266
            n188 = Empty String/Path? "空地址？"(string/path=w262) -> ()  [unwired: 1 out]
            n189 = property on="地址" class="Str"("Caption.Text"=w264, "DisabledEnum"=w263) -> ()  [unwired: 2 in, 2 out]
            n190 = Wait (ms)(milliseconds to wait=u32 10 ("等待时间（毫秒）")) -> ()  [unwired: 1 out]
          }
          event "端口": Value Change {
            # "在串口模式下, 端口是探头编号, 所以要防止冲突"
            n191 = event-data() -> ("NewVal"=w300:u16)  [unwired: 1 in, 5 out]
            n192 = local read "专用标志-首次 '端口值改变' 事件"() -> (w290:bool)
            n193 = case shown="\"串口探头\"" "类型" {
              tunnel: w300 -> [w309 w335]
              tunnel: ["端口 *" ("标题.文本") "探头号 *" ("标题.文本")] -> w298
              tunnel: [w309 w317] -> w297
              tunnel: [w303 w316] -> w285
              tunnel: [_ w318] -> w296
              tunnel: [_ w319] -> w295
              tunnel: w290 -> [w304 w315]
              tunnel: [w308 _] -> w289
              tunnel: [w301 w312] -> w288
              frame "网络探头", Default {
                w308 = FALSE  # F
                # "打开弹窗后, 首次定位到名称\n以后不要"
                n194 = local read "探头属性 i"() -> (w307:T1)
                n195 = Unbundle By Name(w307) -> ("探头地址与信息.网络地址"=w306:string)
                n196 = Empty String/Path?(string/path=w306) -> (empty?=w305:bool)
                n197 = Compound Arithmetic op=AND ("复合运算")(w305, w304) -> (w302:bool)
                n198 = property on="地址" class="Str"("Key Focus"=w302) -> ()  [unwired: 2 in, 2 out]
                n199 = Not(x=w304) -> (.not. x?=w303:bool)
                n200 = Not(x=w302) -> (.not. x?=w301:bool)
              }
              frame "串口探头" {
                w323 = T17."Disabled and Grayed Out" ("禁用")
                w320 = 枚举-配置文件动作."读取配置"  # 读取配置
                w336 = enum16{"新建设备", "编辑设备"}."编辑设备"  # 编辑设备
                # "调试模式下倾向于改地址,\n用户模式下不能改地址"
                # "编辑模式下不用过滤冲突\n用默认值"
                # "检查探头号是否冲突, 自动定位到最近的可用地址"
                n201 = local read "已保存的探头号"() -> (w338:u16[])
                n202 = Search 1D Array(1D array=w338, element=w335) -> (index of element=w340:i32)  [unwired: 1 in]
                n203 = Less Than 0?(x=w340) -> (x < 0?=w339:bool)
                n204 = Bundle By Name(cluster=T19 {"配置文件动作"=enum."初始化加载配置", "数据输入"=variant} ("输入"), "配置文件动作"=w320) -> (w326:T19)
                n205 = case shown="假" w339 {
                  tunnel: [w343 w351] -> w334
                  tunnel: w335 -> [_ w351]
                  tunnel: w338 -> [w344 _]
                  frame False {
                    # "有冲突, 定位到最近的可用地址"
                    n206 = for {
                      N: 255 -> [_]
                      tunnel: w344 -> [w349]
                      tunnel: [w346] -> w343
                      i -> [w350]
                      stop <- w347 stop-if-true
                      # "串口探头, 找出可用的最小地址"
                      n207 = Increment(x=w350) -> (x+1=w346:i32)
                      n208 = Search 1D Array(1D array=w349, element=w346) -> (index of element=w348:i32)  [unwired: 1 in]
                      n209 = Less Than 0?(x=w348) -> (x < 0?=w347:bool)
                    }
                  }
                  frame True {
                    # "可用的地址"
                  }
                }
                n210 = call "TOP-配置文件模块.vi"("输入"=w326) -> ("配置文件"=w325:T21)  [unwired: 9 in, 1 out]
                n211 = Unbundle By Name(w325) -> ("调试模式？"=w311:bool)
                n212 = local read "探头属性 i"() -> (w331:T1)
                n213 = Unbundle By Name(w331) -> ("探头地址与信息.网络地址"=w330:string)
                n214 = call "网络地址字符串 转 IP端口.vi"("IP端口字符串"=w330) -> ("IP端口"=w329:cluster{"IP":string, "Port":u16})  [unwired: 10 in]
                n215 = local read "模式"() -> (w337:enum16{"新建设备", "编辑设备"})
                n216 = Unbundle By Name(w329) -> ("Port"=w328:u16)
                n217 = Equal?(x=w336, y=w337) -> (x = y?=w318:bool)
                n218 = Not(x=w318) -> (.not. x?=w313:bool)
                n219 = Select(t=w335, s=w318, f=w334) -> (s? t:f=w317:i32)
                n220 = Compound Arithmetic op=AND ("复合运算")(w313, w315) -> (w314:bool)
                n221 = case shown="真" w314 {
                  tunnel: w317 -> [_ w342]
                  frame False {
                  }
                  frame True {
                    n222 = Number To Decimal String(number=w342) -> (decimal integer string=w341:string)  [unwired: 1 in]
                    n223 = property on="探头名称" class="Str"("Val(Sgnl)"=w341) -> ()  [unwired: 2 in, 2 out]
                  }
                }
                n224 = And(x=w314, y=w311) -> (x .and. y?=w312:bool)
                n225 = Equal?(x=w328, y=w317) -> (x = y?=w327:bool)
                n226 = control-ref of="设置系数"() -> (w332:refnum<vi>)
                n227 = Select(t=T17."Enabled" ("禁用"), s=w318, f=w323) -> (s? t:f=w324:T17)
                n228 = Select(t=w324, s=w311, f=w323) -> (s? t:f=w319:T17)
                n229 = call "控件启用与禁用.vi"("启用？"=w327, "控件引用"=w332) -> ()  [unwired: 9 in, 1 out]
                n230 = Not(x=w312) -> (.not. x?=w316:bool)
              }
            }
            n231 = Bundle By Name(cluster=T18 {"Selection Start"=0, "Selection End"=0} ("文本.选择"), "Selection End"=u32 1000 ("Selection Start")) -> (w292:T18)
            n232 = local write "专用标志-首次 '端口值改变' 事件"(w289) -> ()
            n233 = property on="设置系数" class="Bool"("Visible"=w296, "DisabledEnum"=w295) -> (error out=w286:errorcluster)  [unwired: 2 in, 1 out]
            n234 = property on="端口" class="DigNum (严格)"("Value"=w297, "Caption.Text"=w298, "DisabledEnum"=w295, "Key Focus"=w285) -> (error out=w294:errorcluster)  [unwired: 2 in, 1 out]
            n235 = Merge Errors(w294, w286) -> (w287:errorcluster)
            n236 = property on="探头名称" class="字符串"(error in=w287, "Key Focus"=w288, "Text.Selection"=w292) -> ()  [unwired: 1 in, 2 out]
          }
          event "探头名称": Value Change {
            # "过滤掉特符号"
            # "实时过滤探头名称格式"
            n237 = event-data() -> ()  [unwired: 1 in, 6 out]
            n238 = call <vilib>:"Trim Whitespace.vi"("string"="探头名称") -> ("trimmed string"=w352:string)  [unwired: 1 in]
            n239 = String Subset(string=w352, length (rest)=64 ("长度（剩余）")) -> (substring=w357:string)  [unwired: 1 in]
            n240 = call "字符串过滤-正则表达式.vi"("正则式（非汉字单字符）"="[~ -.!`\\[\\]\"']", "字符串 i"=w357) -> ("字符串 o"=w353:string)  [unwired: 8 in, 1 out]
            n241 = local write "探头名称"(w353) -> ()
            n242 = Empty String/Path?(string/path=w353) -> (empty?=w359:bool)
            n243 = Not(x=w359) -> (.not. x?=→"有效名称？":bool)
            n244 = Wait (ms)(milliseconds to wait=u32 10 ("等待时间（毫秒）")) -> ()  [unwired: 1 out]
          }
        }
        "输出有效？" <- w93
        "改串口地址?" <- w90
        n245 = case shown="真" w92 {
          frame False {
          }
          frame True {
            n246 = call "cmd启动屏幕键盘.vi"("软键盘开关"=enum16{"关闭", "打开"}."关闭") -> ()  [unwired: 9 in, 2 out]
          }
        }
      }
    }
    frame #2 {
      # "不要在这里执行"
      # "执行数据库操作"
      n247 = local read "输出有效？"() -> (w363:bool)
      n248 = local read "探头属性 i"() -> (w362:T1)
      n249 = case shown="真" w363 {
        tunnel: w362 -> [w364 w390]
        tunnel: [w364 w389] -> w361
        frame False {
          # "输出无效, 检查是否要改串口地址"
          n250 = local read "改串口地址?"() -> (w365:bool)
          n251 = case shown="真" w365 {
            tunnel: w364 -> [_ w370]
            frame False {
              # "不改"
            }
            frame True {
              w376 = 串口动作类型."设置地址"  # 设置地址
              # "改串口地址"
              n252 = Unbundle By Name(w370) -> ("探头地址与信息.网络地址"=w369:string)
              n253 = global read "全局变量-35点监测.vi" "波特率"() -> (w371:enum16{"9600", "19200"})
              n254 = global read "全局变量-35点监测.vi" "COM口"() -> (w372:refnum<visa-resource-name>)
              n255 = call "网络地址字符串 转 IP端口.vi"("IP端口字符串"=w369) -> ("IP端口"=w373:cluster{"IP":string, "Port":u16})  [unwired: 10 in]
              n256 = Unbundle By Name(w373) -> ("Port"=w367:u16)
              n257 = Bundle By Name(cluster=T13 {"COM口"="", "波特率"=enum."9600", "探头地址(U8)"=0} ("串口配置"), "COM口"=w372, "波特率"=w371, "探头地址(U8)"=w367) -> (w374:T13)
              n258 = local read "端口"() -> (w366:u16)
              n259 = Bundle By Name(cluster=T15 {"串口动作类型"=enum."读测量值", "串口配置"={"COM口"="", "波特率"=enum."9600", "探头地址(U8)"=0}, "数据输入"=variant} ("串口模块输入"), "串口动作类型"=w376, "串口配置"=w374, "数据输入"=w366) -> (w377:T15)
              n260 = call "TOP-串口通信模块.vi"("串口模块输入"=w377) -> ("error out"=w368:errorcluster)  [unwired: 9 in, 1 out]
              n261 = case shown="无错误" w368 {
                tunnel: w367 -> [w381 _]
                tunnel: w366 -> [w380 _]
                frame No Error {
                  # "修改失败"
                  n262 = call "创建文本"("原地址"=w381, "新地址"=w380) -> ("Result"=→"附加信息":string)  [unwired: 12 in, 1 out]
                }
                frame Error {
                  # "修改地址成功"
                }
              }
            }
          }
        }
        frame True {
          # "确认执行数据库操作 , 添加新设备"
          n263 = local read "探头名称"() -> (w383:string)
          n264 = local read "类型"() -> (w385:enum16{"网络探头", "串口探头"})
          n265 = local read "模式"() -> (w397:enum16{"新建设备", "编辑设备"})
          n266 = local read "前缀"() -> (w384:enum16{"Net", "Serial"})
          n267 = To Unsigned Word Integer(number=w385) -> (unsigned 16bit integer=w386:u16)
          n268 = local read "地址"() -> (w395:string)
          n269 = local read "端口"() -> (w396:u16)
          n270 = call "Number To Enum.vim"("number"=w386, "enum type"=w384) -> ("number as enum"=w387:enum16{"Net", "Serial"})
          n271 = Format Into String(w387) -> (resulting string=w388:string)  [unwired: 3 in, 1 out]
          n272 = Bundle By Name(cluster=cluster{"IP":string, "Port":u16} {"IP"="", "Port"=0} ("IP端口"), "IP"=w395, "Port"=w396) -> (w394:cluster{"IP":string, "Port":u16})
          n273 = call "设备名称过滤.vi"("前缀"=w388, "字符串 i"=w383) -> ("字符串 o"=w382:string)  [unwired: 9 in]
          n274 = call "IP端口 合并 网络地址字符串.vi"("IP端口"=w394) -> ("IP端口字符串"=w392:string)  [unwired: 10 in]
          n275 = case shown="\"新建设备\", 默认" w397 {
            tunnel: w392 -> [w406 w414]
            tunnel: w382 -> [w405 w413]
            tunnel: "探头备注" -> [w404 w412]
            tunnel: [w398 w411] -> w389
            tunnel: w390 -> [_ w410]
            frame "新建设备", Default {
              w408 = 20000.0  # μSv
              w407 = T2 {"网络地址"="", "名称"="", "备注"="", "累积剂量"=0.0, "累积限值"=0.0, "硬件剂量率限值"=enum."一级限值", "剂量率限值1"=0.0, "剂量率限值2"=0.0, "报警方式"=enum."常报警"}  # 探测器信息-完整
              # "职业照射 : 五年平均每年不超过 20mSv"
              # "用默认值补全其他信部分息"
              n276 = Bundle By Name(cluster=w407, "网络地址"=w406, "名称"=w405, "备注"=w404, "累积剂量"=0.0, "累积限值"=w408, "硬件剂量率限值"=探头剂量率限值选择."一级限值", "剂量率限值1"=0.5, "剂量率限值2"=10.0 ("剂量率限值1"), "报警方式"=报警方式选择."常报警") -> (w399:T2)
              n277 = call "用探测器信息 初始化 探头属性.vi"("探测器信息"=w399) -> ("探头属性"=w398:T1)  [unwired: 10 in]
            }
            frame "编辑设备" {
              # "只改变编辑过的部分 , 保留原有其他信息"
              n278 = Bundle By Name(cluster=w410, "探头地址与信息.网络地址"=w414, "探头地址与信息.名称"=w413, "探头地址与信息.备注"=w412) -> (w411:T1)
            }
          }
        }
      }
      "探头属性 o" <- w361
    }
    frame #3 {
      # "结束"
      n279 = invoke class="VI" method="FP.Close"(reference=w415) -> ()  [unwired: 2 in, 3 out]
    }
  }
  "error out" <- "错误输出"
